vi "issues.get.vi"(8 "error in (no error)":errorcluster, 10 "volume ID":i32, 11 "manager_daemon in":refnum<class "manager_daemon.lvclass">) -> (0 "error out":errorcluster, 2 "issues":T1[](array[typedef]), 3 "manager_daemon out":refnum<class "manager_daemon.lvclass">)   [LabVIEW 2024, in "manager_daemon.lvclass"]
uses:
  manager_daemon.lvclass
  manager_daemon.lvclass/manager_daemon.ctl
  type_defs/cmd--enum.ctl
  type_defs/msg--cluster.ctl
  type_defs/IssueData--clustrer.ctl
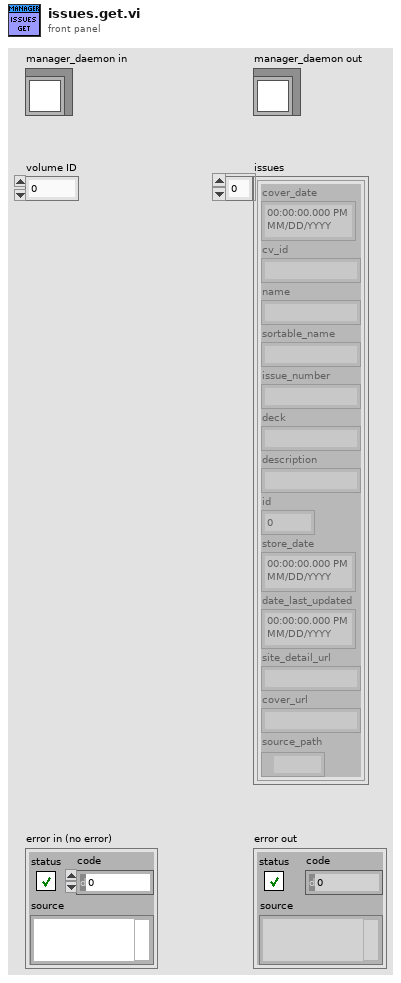
[diagram p1: front panel]
types:
  T1 = typedef "manager_daemon.lvclass/IssueData--clustrer.ctl" = cluster{"cover_date":timestamp, "cv_id":string, "name":string, "sortable_name":string, "issue_number":string, "deck":string, "description":string, "id":i32, "store_date":timestamp, "date_last_updated":timestamp, "site_detail_url":string, "cover_url":string, "source_path":path}
  T2 = typedef "manager_daemon.lvclass/cmd--enum.ctl" = enum16{"init", "run", "load binaries", "build binaries", "save binaries", "create folder map", "display info", "apply filter", "add volume", "add issues", "add issue", "get issues", "get volume", "delete volume", "delete issues", "exit"}
  T3 = typedef "manager_daemon.lvclass/msg--cluster.ctl" = cluster{"cmd":T2, "data":variant}
  T4 = cluster{"volume ID":i32, "notifier out":refnum<notifier>}
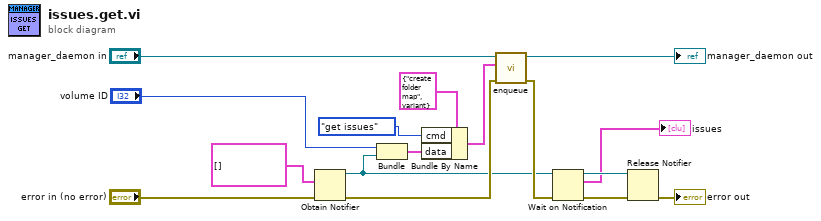
[diagram p0: block diagram]
diagram:
  n1 = Obtain Notifier(notification data type=T1[] [] ("Array"), error in (no error)="error in (no error)") -> (notifier out=w3:refnum<notifier>, error out=w6:errorcluster)  [unwired: 2 in, 1 out]
  n2 = Bundle("volume ID"="volume ID", "notifier out"=w3) -> (w4:T4)  [unwired: 1 in]
  n3 = Bundle By Name(cluster=T3 {"cmd"=enum."create folder map", "data"=variant} ("msg"), "cmd"=cmd--enum."get issues", "data"=w4) -> (w14:T3)
  n4 = call "enqueue.vi"("error in (no error)"=w6, "msg"=w14, "manager_daemon in"="manager_daemon in") -> ("error out"=w13:errorcluster, "manager_daemon out"=→"manager_daemon out":refnum<class "manager_daemon.lvclass">)  [unwired: 7 in]
  n5 = Wait on Notification(notifier=w3, error in (no error)=w13) -> (notifier out=w11:refnum<notifier>, notification=→"issues":T1[], error out=w10:errorcluster)  [unwired: 2 in, 1 out]
  n6 = Release Notifier(notifier=w11, error in (no error)=w10) -> (error out=→"error out":errorcluster)  [unwired: 1 in, 2 out]
